vi "RichToFlatcif_manager_RegisterPluginLoaderRequest.vi"(5 "OutputClusterType":T1, 11 "InputCluster":T4) -> (3 "OutputCluster":T1)   [LabVIEW 2021, in "CIF_Manager_server.lvlib"]
uses:
  CIF_Manager_server.lvlib
  cif_manager_RegisterPluginLoaderRequest.ctl
  cif_manager_LoaderInfoFull.ctl
  cif_manager_LoaderType.ctl
  cif_manager_RegisterPluginLoaderRequest_Flat.ctl
  cif_manager_LoaderInfoFull_Flat.ctl
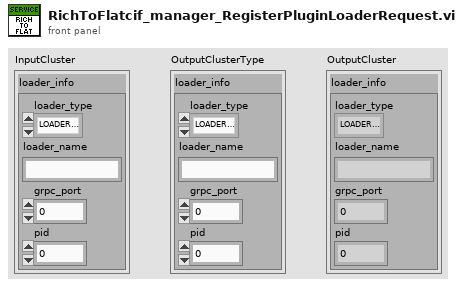
[diagram p1: front panel]
types:
  T1 = typedef "CIF_Manager_server.lvlib/cif_manager_RegisterPluginLoaderRequest_Flat.ctl" = cluster{"loader_info":T2}
  T2 = typedef "CIF_Manager_server.lvlib/cif_manager_LoaderInfoFull_Flat.ctl" = cluster{"loader_type":T3, "loader_name":string, "grpc_port":i32, "pid":u32}
  T3 = typedef "CIF_Manager_server.lvlib/cif_manager_LoaderType.ctl" = enum32{"LOADERTYPE_UNKNOWN", "LOADERTYPE_LABVIEW"}
  T4 = typedef "CIF_Manager_server.lvlib/cif_manager_RegisterPluginLoaderRequest.ctl" = cluster{"loader_info":T5}
  T5 = typedef "CIF_Manager_server.lvlib/cif_manager_LoaderInfoFull.ctl" = cluster{"loader_type":T3, "loader_name":string, "grpc_port":i32, "pid":u32}
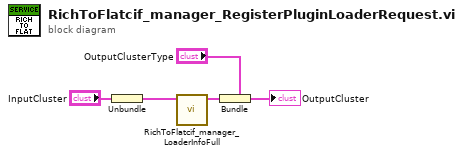
[diagram p0: block diagram]
diagram:
  n1 = Unbundle "Unbundle"("InputCluster") -> ("loader_info"=w2:T5)
  n2 = call "RichToFlatcif_manager_LoaderInfoFull.vi"("InputCluster"=w2) -> ("OutputCluster"=w1:T2)  [unwired: 10 in]
  n3 = Bundle "Bundle"(cluster="OutputClusterType", "loader_info"=w1) -> (→"OutputCluster":T1)
